vi "Do Request.vi"(7 "Processing In":refnum<class "Processing.lvclass">, 11 "StandardFileServe in":refnum<class "StandardFileServe.lvclass">) -> (0 "error out":errorcluster, 5 "Processing":refnum<class "Processing.lvclass">)   [LabVIEW 2020, in "HTTP Server.lvlib" / "StandardFileServe.lvclass"]
uses:
  StandardFileServe.lvclass
  Processing/Processing.lvclass
  Processing/Processing.lvclass/Processing.ctl
  lv-http-util/HTTP Utils/File Response/File Response.lvclass
  C:/dev/lv20CE/relink/lv-http-util/HTTP Utils/Response/Response.lvclass
  StandardFileServe.lvclass/StandardFileServe.ctl
  lv-http-util/HTTP Utils/Request/Request.lvclass
  lv-uri/URI/URI/URI.lvclass
  C:/dev/lv20CE/relink/lv-http-util/HTTP Utils/Streamable Response/Streamable Response.lvclass
  C:/dev/lv20CE/relink/lv-http-util/HTTP Utils/File Response/File Response.lvclass
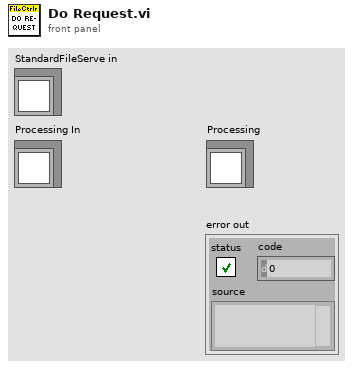
[diagram p1: front panel]
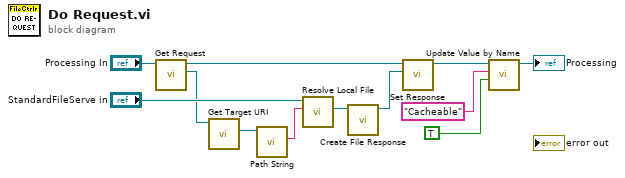
[diagram p0: block diagram]
diagram:
  n1 = call "Get Request.vi"("Processing in"="Processing In") -> ("Request"=w8:refnum<class "Request.lvclass">, "Processing out"=w7:refnum<class "Processing.lvclass">)  [unwired: 9 in]
  n2 = call "Get Target URI.vi"("Request in"=w8) -> ("Target URI"=w12:refnum<class "URI.lvclass">)  [unwired: 8 in, 2 out]
  n3 = call "Path String.vi"("URI in"=w12) -> ("Path String"=w10:string)  [unwired: 9 in, 1 out]
  n4 = call "Resolve Local File.vi"("Request Path"=w10, "StandardFileServe in"="StandardFileServe in") -> ("Path"=w6:path)  [unwired: 7 in, 2 out]
  n5 = call "Create File Response.vi"("Path"=w6) -> ("File Response out"=w5:refnum<class "File Response.lvclass">)  [unwired: 9 in, 1 out]
  n6 = call "Set Response.vi"("Response"=w5, "Processing in"=w7) -> ("Processing out"=w4:refnum<class "Processing.lvclass">)  [unwired: 9 in]
  n7 = call "Update Value by Name.vi"("Value"=TRUE, "Name"="Cacheable", "Processing in"=w4) -> ("Processing out"=→"Processing":refnum<class "Processing.lvclass">)  [unwired: 7 in, 1 out]
